vi "Wrap Angle.vi"   [LabVIEW 2020, in "NI_AAL_Angle.lvlib"]
doc: "Wraps the input angle to a value within the range you specify with <B>angle range</B>.\n\nWire data to any of the angle inputs to determine the polymorphic instance to use or manually select the instance."
uses:
  <vilib>/Analysis/NI_AAL_Angle.lvlib
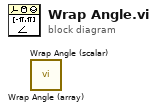
[diagram p0: block diagram]
diagram:
  n1 = call <vilib>:"Wrap Angle (array).vi"() -> ()  [unwired: 10 in, 2 out]
  n2 = call <vilib>:"Wrap Angle (scalar).vi"() -> ()  [unwired: 10 in, 2 out]
